vi "Plot_Beam_Powers.vi"() -> ()   [LabVIEW 2016]
panel:
  in  "Delete First Rows?":bool
  out "XY Graph":cluster{dbl[], dbl[]}[](graph)
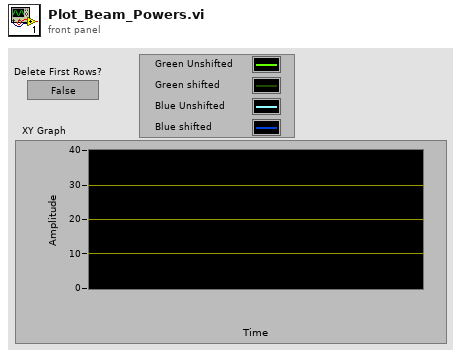
[diagram p1: front panel]
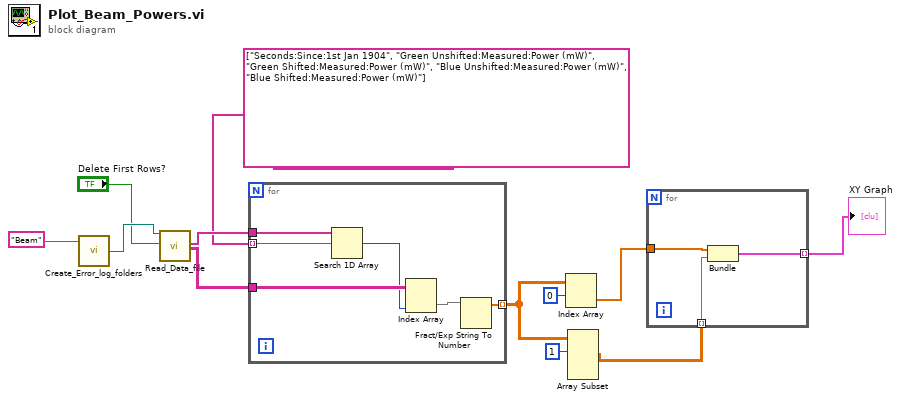
[diagram p0: block diagram]
diagram:
  n1 = call "Create_Error_log_folders.vi"("Log Filename"="Beam" ("Input Element")) -> ("Server copy Location"=w2:path)  [unwired: 2 in, 2 out]
  n2 = call "Read_Data_file.vi"("Results file"=w2, "Delete First Rows?"="Delete First Rows?") -> ("Ch names Out"=w12:string[], "Channel Values Out"=w10:string[][])  [unwired: 7 in, 9 out]
  n3 = for {
    tunnel: w12 -> [w18]
    tunnel: string[] ["Seconds:Since:1st Jan 1904", "Green Unshifted:Measured:Power (mW)", "Green Shifted:Measured:Power (mW)", "Blue Unshifted:Measured:Power (mW)", "Blue Shifted:Measured:Power (mW)"] ("Ch names Out") -> [w17] mode=indexing
    tunnel: w10 -> [w16]
    tunnel: [w13] -> w7 mode=indexing
    n4 = Search 1D Array(1D array=w18, element=w17) -> (index of element=w14:i32)  [unwired: 1 in]
    n5 = Index Array(array=w16, index (col)=w14) -> (element=w15:string[])  [unwired: 1 in]
    n6 = Fract/Exp String To Number(string=w15) -> (number=w13:dbl[])  [unwired: 3 in, 1 out]
  }
  n7 = Index Array(array=w7, index (row)=0) -> (element=w8:dbl[])  [unwired: 1 in]
  n8 = Array Subset(array=w7, index (row)=1 ("index")) -> (w5:dbl[][])  [unwired: 3 in]
  n9 = for {
    tunnel: w8 -> [w21]
    tunnel: w5 -> [w20] mode=indexing
    tunnel: [w19] -> w4 mode=indexing
    n10 = Bundle(w21, w20) -> (w19:cluster{dbl[], dbl[]})  [unwired: 1 in]
  }
  "XY Graph" <- w4
